vi "generarNumeroMayor50subvi.vi"() -> (3 "Numeric":i32)   [LabVIEW 2011]
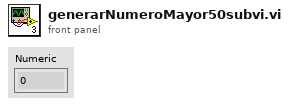
[diagram p1: front panel]
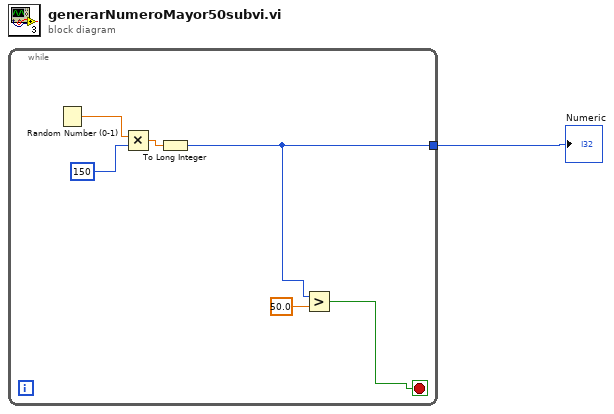
[diagram p0: block diagram]
diagram:
  n1 = while {
    tunnel: [w2] -> w1
    stop <- w4 stop-if-true
    n2 = Random Number (0-1)() -> (number: 0 to 1=w7:dbl)
    n3 = Multiply(x=w7, y=150) -> (x*y=w5:dbl)
    n4 = To Long Integer(number=w5) -> (32bit integer=w2:i32)
    n5 = Greater?(x=w2, y=50.0) -> (0:w4:bool)
  }
  "Numeric" <- w1
